vi "queryAndFetch.vi"(8 "Error In":errorcluster, 10 "Query":string, 11 "DB File Path":path) -> (0 "Error Out":errorcluster, 3 "Result Table":string[][](array[string]))   [LabVIEW 2018]
uses:
  controls/sqlDriverSelectionEnum.ctl
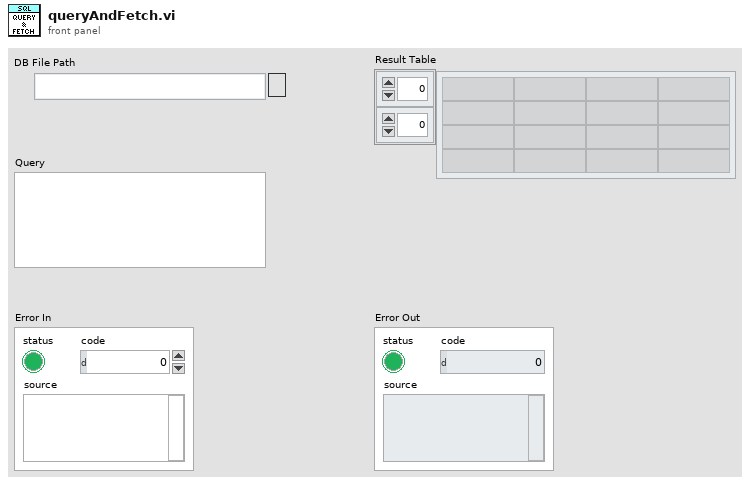
[diagram p1: front panel]
types:
  T1 = typedef "sqlDriverSelectionEnum.ctl" = enum16{"open", "query & fetch", "close"}
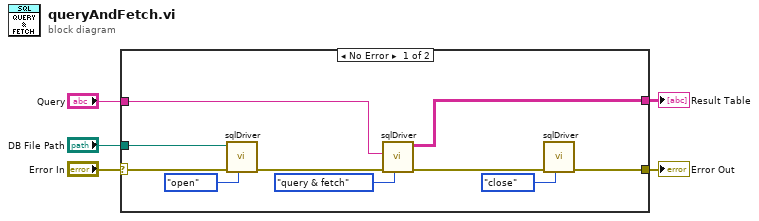
[diagram p0: block diagram]
diagram:
  n1 = case shown="No Error" "Error In" {
    selector: "Error In" -> [w15 w16]
    tunnel: [w10 w16] -> w4
    tunnel: "DB File Path" -> [w13 _]
    tunnel: "Query" -> [w7 _]
    tunnel: [w8 _] -> w2
    frame No Error {
      n2 = call "sqlDriver.vi"("SQL Driver Selection Driver"=sqlDriverSelectionEnum."open", "Error In"=w15, "Database File Path"=w13) -> ("Error Out"=w12:errorcluster)  [unwired: 7 in, 1 out]
      n3 = call "sqlDriver.vi"("SQL Driver Selection Driver"=sqlDriverSelectionEnum."query & fetch", "Error In"=w12, "Query"=w7) -> ("Error Out"=w11:errorcluster, "Result Table"=w8:string[][])  [unwired: 7 in]
      n4 = call "sqlDriver.vi"("SQL Driver Selection Driver"=sqlDriverSelectionEnum."close", "Error In"=w11) -> ("Error Out"=w10:errorcluster)  [unwired: 8 in, 1 out]
    }
    frame Error {
    }
  }
  "Error Out" <- w4
  "Result Table" <- w2
